vi "Get Description.vi"(0 "serial arm in":refnum<class "NI_Robotics_Serial Robot Arm.lvclass">, 11 "error in (no error)":errorcluster) -> (4 "serial arm out":refnum<class "NI_Robotics_Serial Robot Arm.lvclass">, 6 "name":string, 8 "manufacturer":string, 10 "comment":string, 15 "error out":errorcluster)   [LabVIEW 2017, in "NI_Robotics_Serial Robot Arm.lvclass"]
uses:
  <vilib>/robotics/Kinematics/Robot/NI_Robotics_Serial Robot Arm.lvclass
  <vilib>/robotics/Kinematics/Robot/NI_Robotics_Serial Robot Arm.lvclass/NI_Robotics_Serial Robot Arm.ctl
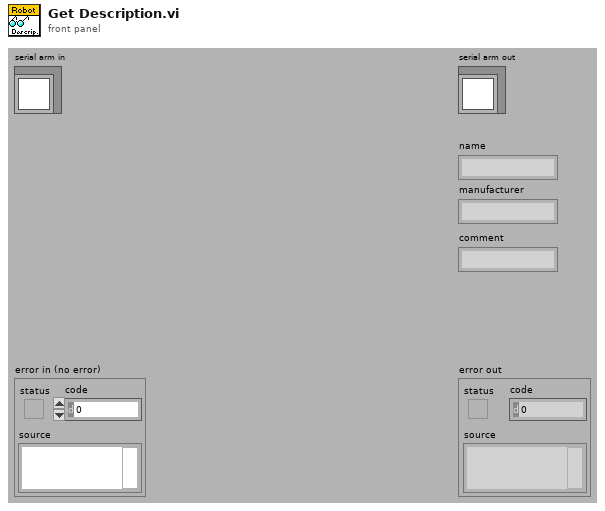
[diagram p1: front panel]
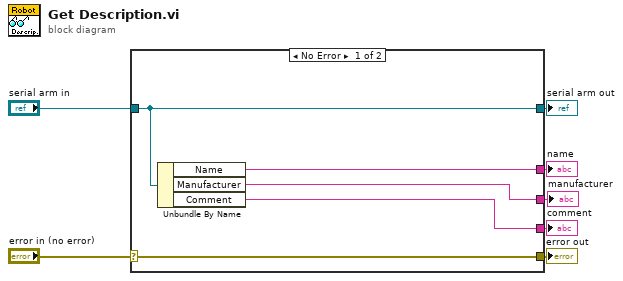
[diagram p0: block diagram]
diagram:
  n1 = case shown="No Error" "error in (no error)" {
    selector: "error in (no error)" -> [w12 w13]
    tunnel: [w12 w13] -> w6
    tunnel: [w11 w14] -> w4
    tunnel: "serial arm in" -> [w11 w14]
    tunnel: [w10 _] -> w3
    tunnel: [w9 _] -> w2
    tunnel: [w8 _] -> w1
    frame No Error {
      n2 = Unbundle By Name(w11) -> ("Name"=w10:string, "Manufacturer"=w9:string, "Comment"=w8:string)
    }
    frame Error {
    }
  }
  "error out" <- w6
  "serial arm out" <- w4
  "name" <- w3
  "manufacturer" <- w2
  "comment" <- w1
